vi "Set Environment Variable.vi"   [LabVIEW 2011]
uses:
  <vilib>/registry/registry.llb/Registry RtKey.ctl
  <vilib>/registry/registry.llb/Write Registry Value Simple STR.vi
types:
  T1 = typedef "Registry RtKey.ctl" = enum32{"HKEY_CLASSES_ROOT", "HKEY_CURRENT_USER", "HKEY_LOCAL_MACHINE", "HKEY_USERS", "HKEY_PERFORMANCE_DATA", "HKEY_CURRENT_CONFIG", "HKEY_DYN_DATA"}
  T2 = typedef "Registry refnum.ctl" = refnum<k1>
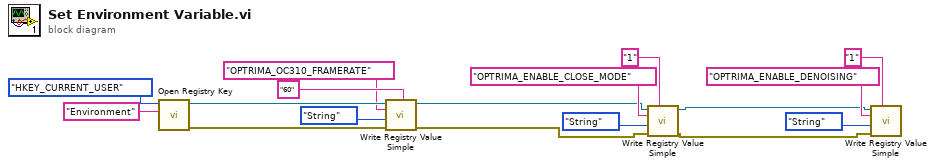
[diagram p0: block diagram]
diagram:
  n1 = call <vilib>:"Open Registry Key.vi"("subkey"="Environment", "root key (HKEY_LOCAL_MACHINE)"=Registry_RtKey."HKEY_CURRENT_USER") -> ("error out"=w11:errorcluster, "refnum out"=w14:T2)  [unwired: 8 in]
  n2 = call-poly <vilib>:"Write Registry Value Simple.vi"("String/Binary data"="60" ("Variable Value"), "error in (no error)"=w11, "simple data type"=enum16{"String", "Binary", "DWORD"}."String", "value"="OPTRIMA_OC310_FRAMERATE" ("Variable Name"), "refnum"=w14) -> ("error out"=w8:errorcluster, "refnum out"=w7:T2)  [unwired: 3 in]
  n3 = call-poly <vilib>:"Write Registry Value Simple.vi"("String/Binary data"="1", "error in (no error)"=w8, "simple data type"=enum16{"String", "Binary", "DWORD"}."String", "value"="OPTRIMA_ENABLE_CLOSE_MODE" ("Variable Name"), "refnum"=w7) -> ("error out"=w2:errorcluster, "refnum out"=w1:T2)  [unwired: 3 in]
  n4 = call-poly <vilib>:"Write Registry Value Simple.vi"("String/Binary data"="1", "error in (no error)"=w2, "simple data type"=enum16{"String", "Binary", "DWORD"}."String", "value"="OPTRIMA_ENABLE_DENOISING" ("Variable Name"), "refnum"=w1) -> ()  [unwired: 3 in, 2 out]
